vi "FPGA Phasor Measurement for P Class.vi"   [LabVIEW 2013, in "NI_EP_PMU_FPGA.lvlib"]
doc: "Calculates the instantaneous magnitude, phase, and frequency values of the fundamental frequency component as defined in the P class of performance in IEEE Std C37.118.1-2011. This VI resamples even-time-spaced voltage and current signals into even-angle-spaced signals. The input signals must have a sample rate of 50 kHz. The output rate is 25 samples per cycle. You must manually select the polymorphic instance to use."
uses:
  <vilib>/addons/Electrical Power/PMU/NI_EP_PMU_FPGA.lvlib
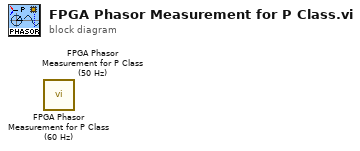
[diagram p0: block diagram]
diagram:
  n1 = call <vilib>:"FPGA Phasor Measurement for P Class (60 Hz).vi"() -> ()  [unwired: 12 in, 4 out]
  n2 = call <vilib>:"FPGA Phasor Measurement for P Class (50 Hz).vi"() -> ()  [unwired: 12 in, 4 out]
